vi "Meas_Two_Edge_Separation-Buffered-Finite.vi"() -> ()   [LabVIEW 2014]
doc: "I. Description:\nThis example demonstrates how to perform a finite number of two edge separation measurements on a Counter Input Channel. The First Edge, Second Edge, Minimum Value, Maximum Value, and Samples to Read are all configurable. \n\nThis example shows how to perform a two edge separation measurement on the counter's default input terminals (refer to section IV, I/O Connections Overview, below for more information), but could easily be expanded to measure two edge separation on any PFI, RTSI, or internal signal.\n\nRefer to your device documentation to see if your device supports two edge separation measurements.\n\nII. Instructions for Running:\n1. Select the Physical Channel which corresponds to the counter on the DAQ device you want to perform a two edge separation measurement on.\n2. Enter the First Edge and Second Edge corresponding to the two edges you want the counter to measure. Enter the Maximum and Minimum Value to specify the range of your unknown two edge separation. Additionally, you can change the First and Second Edge Input Terminals using the channel property node.\nNote: It is important to set the Maximum and Minimum Values of your unknown two edge separation as accurately as possible so the best internal timebase can be chosen to minimize measurement error. The default values specify a range that can be measured by the counter using the 20MHzTimebase.\n3. Set the Samples to Read control. This will determine how many samples are read each time the while loop iterates.\n\nIII. Block Diagram Steps:\n1. Create a Counter Input channel to perform a Two Edge Separation measurement. The First and Second Edge parameters are used to specify the rising or falling edge of one digital signal and the rising or falling edge of another digital signal. It is important to set the Maximum and Minimum Values of your unknown two edge separation as accurately as possible so the best internal timebase can be chosen to minimize measurement error. The default values specify a range that can be measured by the counter using the 20MHzTimebase.\n2. Call the DAQmx Timing VI (Implicit) to configure the Sample Mode and Samples per Channel. Note: For time measurements with counters, the implicit timing VI is used because the signals being measured determine the sample rate. \n3. Call the Start VI to arm the counter and begin measuring.\n4. For finite measurements, the counter will stop reading data when the Samples per Channel have been received. \n5. Call the Clear Task VI to clear the Task.\n6. Use the popup dialog box to display an error if any.\n\nIV. I/O Connections Overview:\nThe counter will perform a two edge separation measurement on the First and Second Edge Input Terminals of the counter specified in the Physical Channel I/O control. \n\n In this example the two edge separation will be measured on the default input terminals on ctr0. \n\nFor more information on the default counter input and output terminals for your device, open the NI-DAQmx Help, and refer to Counter Signal Connections found under the Device Considerations book in the table of contents."
uses:
  <vilib>/Utility/error.llb/DialogType.ctl
  <vilib>/DAQmx/create/channels.llb/DAQmx Create Channel (CI-Two Edge Separation).vi
  <vilib>/DAQmx/configure/timing.llb/DAQmx Timing (Implicit).vi
  <vilib>/DAQmx/read.llb/DAQmx Read (Counter DBL 1Chan 1Samp).vi
panel:
  out "Data (sec)":dbl caption="Waveform" format="%0.9f"
  in  "Second Edge":i32(ring)=10280 items=["Rising"=10280, "Falling"=10171]
  in  "First Edge":i32(ring)=10280 items=["Rising"=10280, "Falling"=10171]
  in  "Counter(s)":tag="Dev1/ctr0" caption="Counter"
  in  "Minimum Value (sec)":dbl=1e-05 format="%0.9f"
  in  "Maximum Value (sec)":dbl=0.005 format="%0.9f"
  in  "Samples per Channel":i32=1
  # "For instructions, select Help>>Show Context Help"
  # "Channel Parameters"
  # "Timing Parameters"
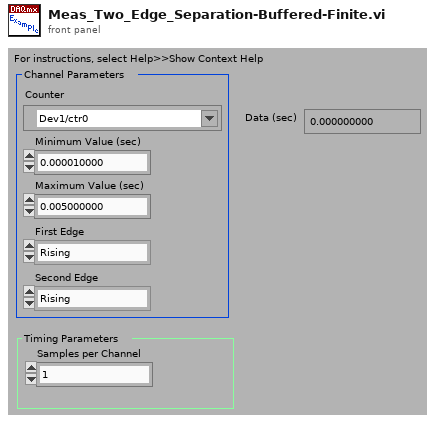
[diagram p1: front panel]
types:
  T1 = typedef "DialogType.ctl" = u16
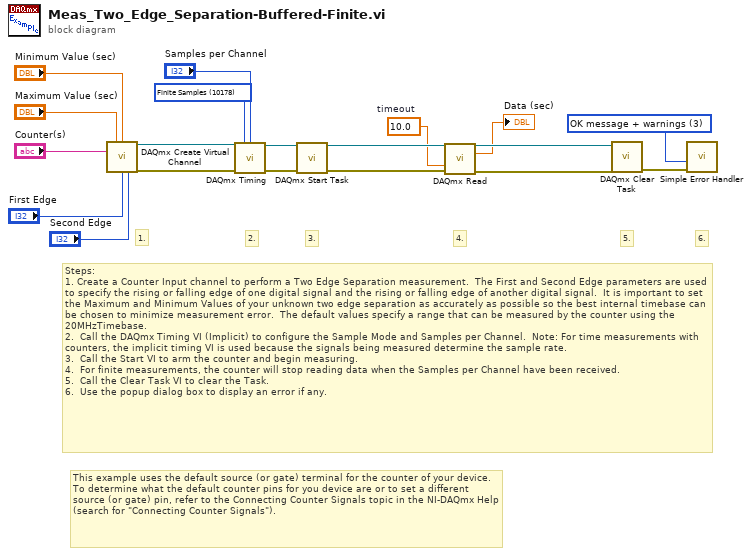
[diagram p0: block diagram]
diagram:
  w4 = T1 3 items=["no dialog", "OK message", "continue or stop message", "OK message + warnings", "continue/stop + warnings"] ("type of dialog (OK msg:1)")
  w5 = 10178 items=["Finite Samples"=10178, "Continuous Samples"=10123] ("sample mode")
  w7 = 10.0  # timeout
  # "This example uses the default source (or gate) terminal for the counter of your device.  To determine what the default counter pins for you device are or to set a different source (or gate) pin, refer to the Connecting Counter Signals topic in the NI-DAQmx Help (search for \"Connecting Counter Signals\")."
  # "4."
  # "6."
  # "3."
  # "2."
  # "Steps: \n1. Create a Counter Input channel to perform a Two Edge Separation measurement.  The First and Second Edge parameters are used to specify the rising or falling edge of one digital signal and the rising or falling edge of another digital signal.  It is important to set the Maximum and Minimum Values of your unknown two edge separation as accurately as possible so the best internal timebase can be chosen to minimize measurement error.  The default values specify a range that can be measured by the counter using the 20MHzTimebase.\n2.  Call the DAQmx Timing VI (Implicit) to configure the Sample Mode and Samples per Channel.  Note: For time measurements with counters, the implicit timing VI is used because the signals being measured determine the sample rate. \n3.  Call the Start VI to arm the counter and begin measuring.\n4.  For finite measurements, the counter will stop reading data when the Samples per Channel have been received.  \n5.  Call the Clear Task VI to clear the Task.\n6.  Use the popup dialog box to display an error if any."
  # "5."
  # "1."
  n1 = call-poly <vilib>:"DAQmx Create Virtual Channel.vi"("maximum value"="Maximum Value (sec)", "minimum value"="Minimum Value (sec)", "counter"="Counter(s)", "first edge"="First Edge", "second edge"="Second Edge") -> ("task out"=w12:refnum<k21>, "error out"=w13:errorcluster)  [unwired: 9 in]
  n2 = call-poly <vilib>:"DAQmx Timing.vi"("task/channels in"=w12, "sample mode"=w5, "samples per channel"="Samples per Channel", "error in"=w13) -> ("task out"=w15:refnum<k21>, "error out"=w16:errorcluster)  [unwired: 10 in]
  n3 = call <vilib>:"DAQmx Start Task.vi"("task/channels in"=w15, "error in"=w16) -> ("task out"=w17:refnum<k21>, "error out"=w18:errorcluster)  [unwired: 12 in]
  n4 = call-poly <vilib>:"DAQmx Read.vi"("task/channels in"=w17, "timeout"=w7, "error in"=w18) -> ("task out"=w11:refnum<k21>, "data"=→"Data (sec)":dbl, "error out"=w6:errorcluster)  [unwired: 10 in]
  n5 = call <vilib>:"DAQmx Clear Task.vi"("task in"=w11, "error in"=w6) -> ("error out"=w19:errorcluster)  [unwired: 13 in]
  n6 = call <vilib>:"Simple Error Handler.vi"("type of dialog (OK msg:1)"=w4, "error in (no error)"=w19) -> ()  [unwired: 3 in, 5 out]
